vi "Moving Average (multiple).vi"(8 "error in (no error)":errorcluster, 10 "window":dbl, 11 "XY-data":cluster{"X-array":dbl[], "Y-array":dbl[]}[](array[cluster])) -> (0 "error out":errorcluster, 3 "XY-data out":cluster{"X-array":dbl[], "Y-array":dbl[]}[](array[cluster]) {"Y-array" format="%.2p"; "X-array" format="%.2p"})   [LabVIEW 2019, in "xy_utilities.lvlib"]
doc: "Apply a moving average <b>XY-data</b>'s Y-Array according to <b>window</b>\n\nWire data to the data input to determine the polymorphic instance to use or manually select the instance."
uses:
  xy_utilities.lvlib
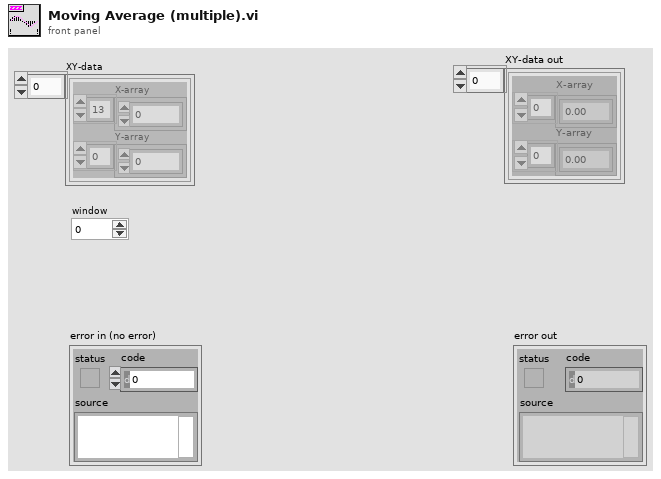
[diagram p1: front panel]
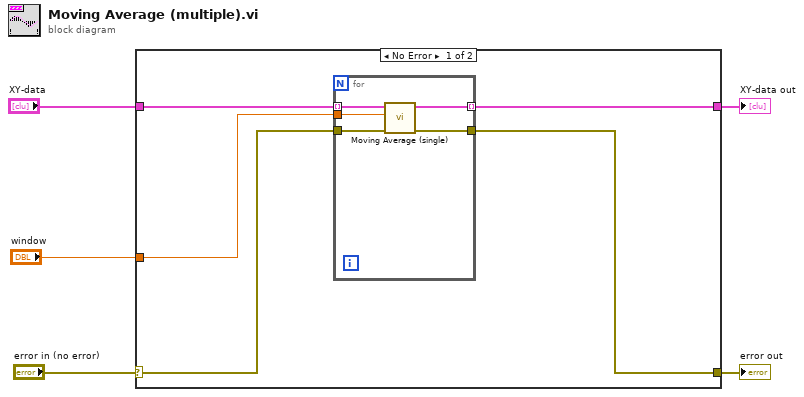
[diagram p0: block diagram]
diagram:
  n1 = case shown="No Error" "error in (no error)" {
    selector: "error in (no error)" -> [w7 w17]
    tunnel: [w6 w17] -> w4
    tunnel: "XY-data" -> [w10 w16]
    tunnel: [w9 w16] -> w2
    tunnel: "window" -> [w8 _]
    frame No Error {
      n2 = for {
        tunnel: w10 -> [w15] mode=indexing
        tunnel: [w14] -> w9 mode=indexing
        tunnel: w8 -> [w13]
        tunnel: w7 -> [w12]
        tunnel: [w11] -> w6
        n3 = call "Moving Average (single).vi"("error in (no error)"=w12, "window"=w13, "XY-data"=w15) -> ("error out"=w11:errorcluster, "XY-data out"=w14:cluster{"X-array":dbl[], "Y-array":dbl[]})  [unwired: 7 in]
      }
    }
    frame Error {
    }
  }
  "error out" <- w4
  "XY-data out" <- w2
